vi "Re-configure Acquisition.vi"(8 "error in (no error)":errorcluster, 10 "Frequency":dbl, 11 "Scope In":refnum<k15>) -> (0 "error out":errorcluster, 3 "Scope out":refnum<k15>)   [LabVIEW 2023, in "Bode Plot - PXI.lvlib"]
doc: "Reconfigures the acquistion, to always acquire ten periods and modifies the vertical range, to use the full dynamic range of the scope"
uses:
  Bode Plot - PXI.lvlib
  <instrlib>/niScope/Controls/niScope vertical coupling.ctl
  <instrlib>/niScope/Acquire/niScope Multi Read WDT.vi
  <vilib>/measure/mascope.llb/Amplitude and Levels 1 chan.vi
  <vilib>/measure/NI_MAPro.lvlib
panel:
  out "32bit integer":i32
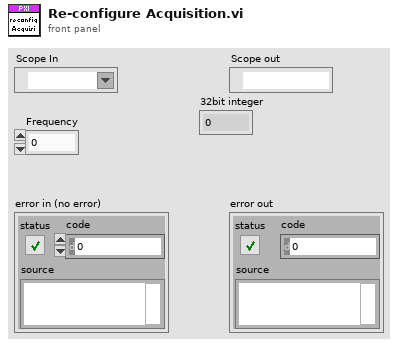
[diagram p1: front panel]
types:
  T1 = typedef "niScope vertical coupling.ctl" = i32
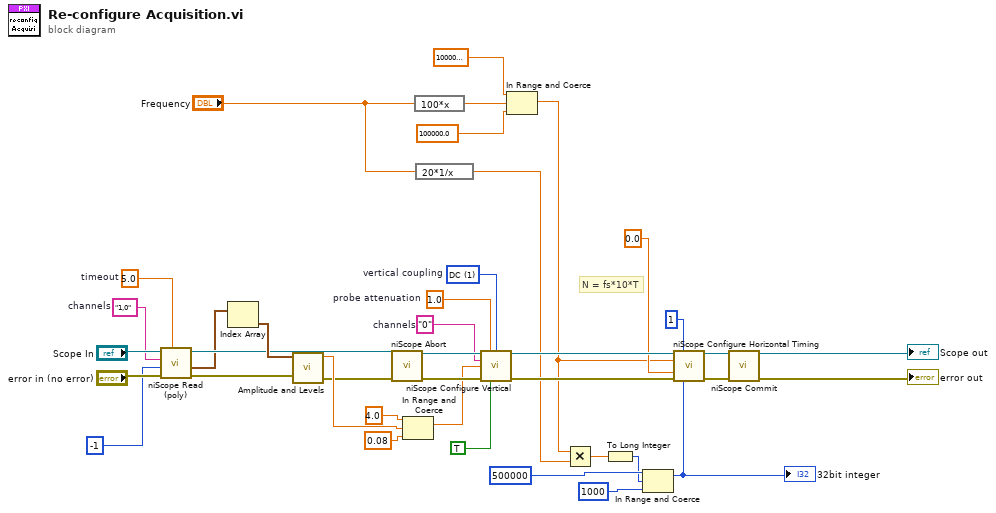
[diagram p0: block diagram]
diagram:
  w11 = 5.0  # timeout
  w12 = T1 1 items=["AC", "DC", "Ground"]  # vertical coupling
  w13 = 1.0  # probe attenuation
  w16 = "0"  # channels
  w17 = "1,0"  # channels
  # "N = fs*10*T"
  n1 = call-poly <instrlib>:"niScope Read (poly).vi"("timeout"=w11, "error in"="error in (no error)", "numSamples"=-1, "channels"=w17, "instrument handle"="Scope In") -> ("error out"=w33:errorcluster, "wfm"=w18:waveform(dbl)[], "instrument handle out"=w30:refnum<k15>)  [unwired: 3 in, 1 out]
  n2 = Index Array(array=w18) -> (element=w32:waveform(dbl))  [unwired: 1 in]
  n3 = call-poly <vilib>:"Amplitude and Levels.vi"("error in (no error)"=w33, "signal in"=w32) -> ("error out"=w29:errorcluster, "amplitude"=w31:dbl)  [unwired: 6 in, 2 out]
  n4 = call <instrlib>:"niScope Abort.vi"("instrument handle"=w30, "error in"=w29) -> ("instrument handle out"=w28:refnum<k15>, "error out"=w27:errorcluster)  [unwired: 12 in]
  n5 = In Range and Coerce(upper limit=4.0, x=w31, lower limit=0.08) -> (coerced(x)=w15:dbl)  [unwired: 1 out]
  n6 = expression code="100*x"("Frequency") -> (w37:dbl)
  n7 = expression code="20*1/x"("Frequency") -> (w6:dbl)
  n8 = call <instrlib>:"niScope Configure Vertical.vi"("instrument handle"=w28, "probe attenuation"=w13, "vertical coupling"=w12, "channels"=w16, "vertical range"=w15, "error in"=w27, "channel enabled"=TRUE) -> ("instrument handle out"=w21:refnum<k15>, "error out"=w20:errorcluster)  [unwired: 7 in]
  n9 = In Range and Coerce(upper limit=100000000.0, x=w37, lower limit=100000.0 ("upper limit")) -> (coerced(x)=w7:dbl)  [unwired: 1 out]
  n10 = Multiply(x=w7, y=w6) -> (x*y=w8:dbl)
  n11 = To Long Integer(number=w8) -> (32bit integer=w4:i32)
  n12 = In Range and Coerce(upper limit=500000, x=w4, lower limit=1000) -> (coerced(x)=w3:i32)  [unwired: 1 out]
  "32bit integer" <- w3
  n13 = call <instrlib>:"niScope Configure Horizontal Timing.vi"("instrument handle"=w21, "number of records"=1, "min sample rate"=w7, "reference position"=0.0, "error in"=w20, "min record length"=w3) -> ("instrument handle out"=w22:refnum<k15>, "error out"=w19:errorcluster)  [unwired: 8 in]
  n14 = call <instrlib>:"niScope Commit.vi"("instrument handle"=w22, "error in"=w19) -> ("instrument handle out"=→"Scope out":refnum<k15>, "error out"=→"error out":errorcluster)  [unwired: 12 in]
